vi "Extract Scaling Info.vi"(8 "Error In":errorcluster, 9 "Validation Set In":T1[](array[typedef]), 10 "Teaching Set In":T1[](array[typedef]), 11 "Neural Network In":T3) -> (0 "Error Out":errorcluster, 1 "Validation Set Out":T1[](array[typedef]), 2 "Teaching Set Out":T1[](array[typedef]), 3 "Neural Network Out":T3)   [LabVIEW 2013, in "Super Simple Neural Network.lvlib"]
uses:
  Super Simple Neural Network.lvlib
  Types/Neural Network.ctl
  Types/2D Array.ctl
  Types/Scaling Info.ctl
  Types/Teaching Vector.ctl
  Types/1D Array.ctl
  MD Select 1D DBL.vi
  Scale Array.vi
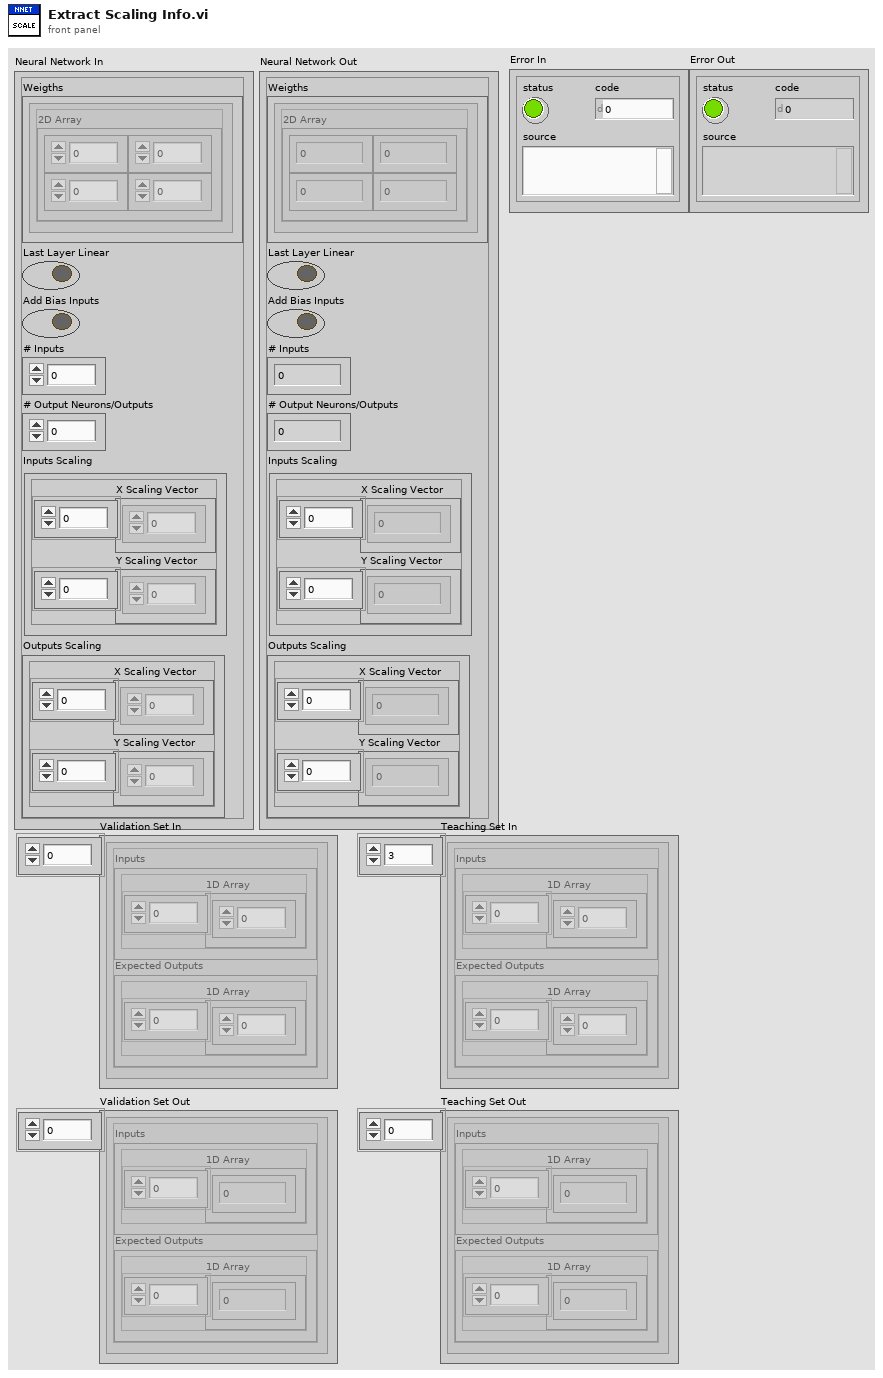
[diagram p1: front panel]
types:
  T1 = typedef "Super Simple Neural Network.lvlib/Teaching Vector.ctl" = cluster{"Inputs":T2, "Expected Outputs":T2}
  T2 = typedef "Super Simple Neural Network.lvlib/1D Array.ctl" = cluster{"1D Array":dbl[]}
  T3 = typedef "Super Simple Neural Network.lvlib/Neural Network.ctl" = cluster{"Weigths":T4[], "Last Layer Linear":bool, "Add Bias Inputs":bool, "# Inputs":u32, "# Output Neurons/Outputs":u32, "Inputs Scaling":T5, "Outputs Scaling":T5}
  T4 = typedef "Super Simple Neural Network.lvlib/2D Array.ctl" = cluster{"2D Array":dbl[][]}
  T5 = typedef "Super Simple Neural Network.lvlib/Scaling Info.ctl" = cluster{"X Scaling Vector":dbl[], "Y Scaling Vector":dbl[]}
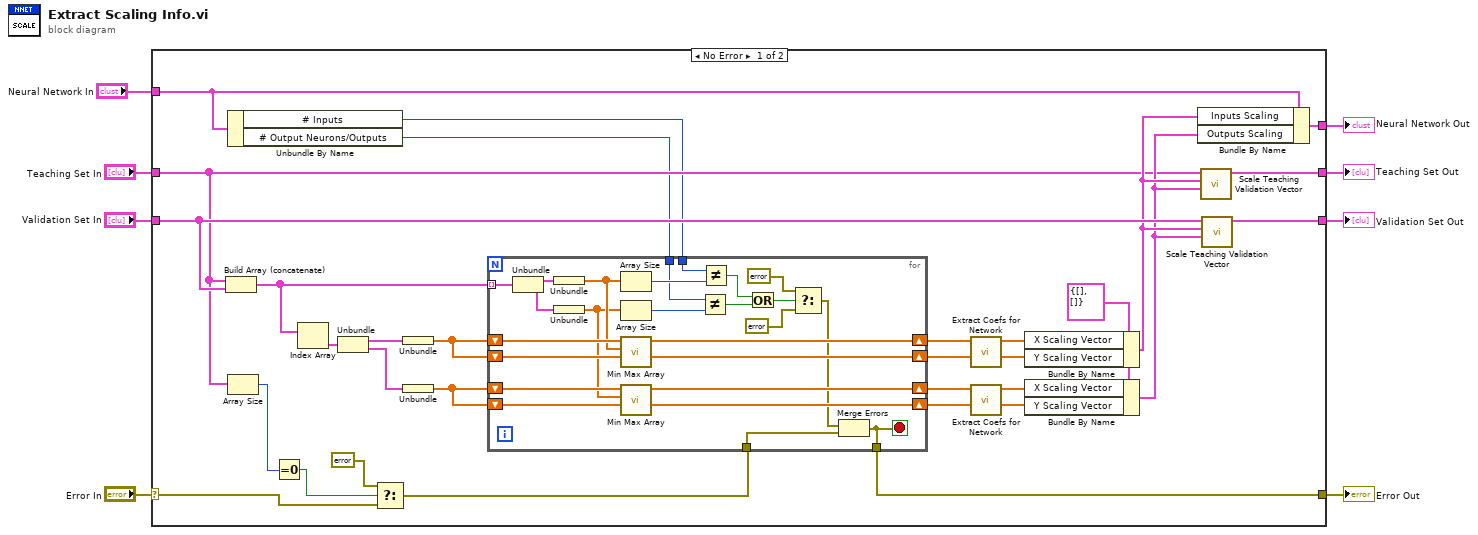
[diagram p0: block diagram]
diagram:
  n1 = case shown="No Error" "Error In" {
    selector: "Error In" -> [w14 w68]
    tunnel: [w29 w67] -> w8
    tunnel: "Validation Set In" -> [w23 w66]
    tunnel: [w22 w66] -> w6
    tunnel: "Neural Network In" -> [w13 w65]
    tunnel: [w21 w65] -> w4
    tunnel: "Teaching Set In" -> [w17 w67]
    tunnel: [w9 w68] -> w2
    frame No Error {
      w26 = T5 {"X Scaling Vector"=[], "Y Scaling Vector"=[]}
      n2 = Build Array (concatenate)(w17, w23) -> (w39:T1[])
      n3 = Unbundle By Name(w13) -> ("# Inputs"=w12:u32, "# Output Neurons/Outputs"=w11:u32)
      n4 = Array Size(array=w17) -> (size(s)=w16:i32)
      n5 = Equal To 0?(x=w16) -> (x = 0?=w15:bool)
      n6 = Index Array(array=w39) -> (element=w36:T1)  [unwired: 1 in]
      n7 = Unbundle(w36) -> ("Inputs"=w37:T2, "Expected Outputs"=w38:T2)
      n8 = Select(t=errorcluster {"status"=TRUE, "code"=5556, "source"="The teaching set cannot be empty."}, s=w15, f=w14) -> (s? t:f=w10:errorcluster)
      n9 = Unbundle(w37) -> ("1D Array"=w35:dbl[])
      n10 = Unbundle(w38) -> ("1D Array"=w34:dbl[])
      n11 = for {
        tunnel: w39 -> [w64] mode=indexing
        shift-right: [w61] -> w30
        shift-left: w35 -> [w58]
        shift-right: [w59] -> w33
        shift-left: w35 -> [w60]
        shift-right: [w55] -> w32
        shift-left: w34 -> [w57]
        shift-right: [w54] -> w31
        shift-left: w34 -> [w56]
        tunnel: w12 -> [w50]
        tunnel: w11 -> [w48]
        tunnel: w10 -> [w42]
        tunnel: [w43] -> w9
        stop <- w43 stop-if-true
        n12 = Unbundle(w64) -> ("Inputs"=w63:T2, "Expected Outputs"=w62:T2)
        n13 = Unbundle(w63) -> ("1D Array"=w53:dbl[])
        n14 = Unbundle(w62) -> ("1D Array"=w51:dbl[])
        n15 = Array Size(array=w53) -> (size(s)=w52:i32)
        n16 = Array Size(array=w51) -> (size(s)=w49:i32)
        n17 = call "Min Max Array.vi"("Min Values"=w60, "Input Array"=w53, "Max Values"=w58) -> ("Min Values Out"=w59:dbl[], "Max Values Out"=w61:dbl[])  [unwired: 7 in]
        n18 = call "Min Max Array.vi"("Min Values"=w56, "Input Array"=w51, "Max Values"=w57) -> ("Min Values Out"=w54:dbl[], "Max Values Out"=w55:dbl[])  [unwired: 7 in]
        n19 = Not Equal?(x=w48, y=w49) -> (x != y?=w47:bool)
        n20 = Not Equal?(x=w50, y=w52) -> (x != y?=w46:bool)
        n21 = Or(x=w46, y=w47) -> (x .or. y?=w45:bool)
        n22 = Select(t=errorcluster {"status"=TRUE, "code"=5557, "source"="The number of inputs or outputs in the teaching vectors is not equal to declared number of inputs and outputs in the network. Correct the teaching set or change the parameters\nof the network."} ("error IO"), s=w45, f=errorcluster {"status"=FALSE, "code"=0, "source"=""} ("error IO")) -> (s? t:f=w41:errorcluster)
        n23 = Merge Errors(w41, w42) -> (w43:errorcluster)
      }
      n24 = call "Extract Coefs for Network.vi"("Min Array"=w33, "Max Array"=w30) -> ("Y Scaling Vector"=w27:dbl[], "X Scaling Vector"=w28:dbl[])  [unwired: 8 in]
      n25 = call "Extract Coefs for Network.vi"("Min Array"=w31, "Max Array"=w32) -> ("Y Scaling Vector"=w24:dbl[], "X Scaling Vector"=w25:dbl[])  [unwired: 8 in]
      n26 = Bundle By Name(cluster=w26, "X Scaling Vector"=w28, "Y Scaling Vector"=w27) -> (w20:T5)
      n27 = Bundle By Name(cluster=w26, "X Scaling Vector"=w25, "Y Scaling Vector"=w24) -> (w19:T5)
      n28 = Bundle By Name(cluster=w13, "Inputs Scaling"=w20, "Outputs Scaling"=w19) -> (w21:T3)
      n29 = call "Scale Teaching Validation Vector.vi"("Output Scaling"=w19, "Input Scaling"=w20, "Teaching/Validation Vector In"=w17) -> ("Scaled Teaching/Validation Vector Out"=w29:T1[])  [unwired: 8 in]
      n30 = call "Scale Teaching Validation Vector.vi"("Output Scaling"=w19, "Input Scaling"=w20, "Teaching/Validation Vector In"=w23) -> ("Scaled Teaching/Validation Vector Out"=w22:T1[])  [unwired: 8 in]
    }
    frame Error {
    }
  }
  "Neural Network Out" <- w4
  "Validation Set Out" <- w6
  "Teaching Set Out" <- w8
  "Error Out" <- w2
